vi "Actor Core.vi"(8 "error in":errorcluster, 11 "Sensor in":refnum<class "Sensor.lvclass">) -> (0 "error out":errorcluster, 3 "Actor out":refnum<class "Actor.lvclass">)   [LabVIEW 2012, in "Sensor Definition.lvlib" / "Sensor.lvclass"]
doc: "(<B>Filename</B>: Actor Framework.lvlib:Actor.lvclass:Actor Core.vi)\n\nReceives messages to the actor, reacts to them, and initiates any error handling that may shut the actor down.\n\nDescendant classes may override this VI to append parallel tasks for the actor to complete while it handles messages. Overrides use the Call Parent Method node."
uses:
  Sensor.lvclass
  <vilib>/ActorFramework/Actor/Actor.lvclass
  SensorCharm.lvclass
  Win8uiFramework/CharmView.lvclass
  <vilib>/ActorFramework/Actor/Actor.lvclass/Actor.ctl
  Sensor.lvclass/Sensor.ctl
  Write Owner.vi
  Read CharmView Actor.vi
  Write CharmView Actor.vi
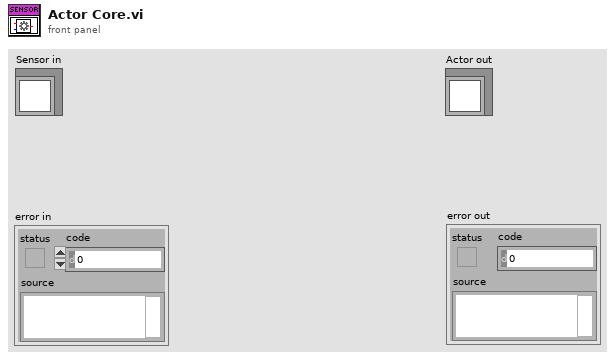
[diagram p1: front panel]
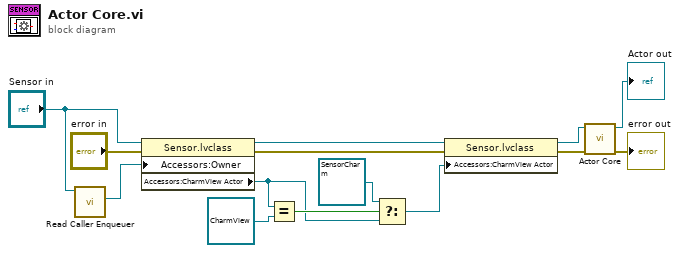
[diagram p0: block diagram]
diagram:
  n1 = call <vilib>:"Read Caller Enqueuer.vi"("Actor"="Sensor in") -> ("Caller Enqueuer"=w10:refnum<class "Message Enqueuer.lvclass">)  [unwired: 10 in]
  n2 = property class="Sensor.lvclass"(reference="Sensor in", error in="error in", "Accessors:Owner"=w10) -> (reference out=w9:refnum<class "Sensor.lvclass">, error out=w8:errorcluster, "Accessors:CharmView Actor"=w3:refnum<class "SensorCharm.lvclass">)
  n3 = Equal?(x=w3, y=refnum<class "CharmView.lvclass"> refnum ("Win8uiFramework.lvlib:CharmView.lvclass")) -> (x = y?=w4:bool)
  n4 = Select(t=refnum<class "SensorCharm.lvclass"> refnum ("Sensor Definition.lvlib:SensorCharm.lvclass"), s=w4, f=w3) -> (s? t:f=w1:refnum<class "SensorCharm.lvclass">)
  n5 = property class="Sensor.lvclass"(reference=w9, error in=w8, "Accessors:CharmView Actor"=w1) -> (reference out=w6:refnum<class "Sensor.lvclass">, error out=w7:errorcluster)
  n6 = call-parent "Actor Core.vi"("error in"=w7, "Actor in"=w6) -> ("error out"=→"error out":errorcluster, "Actor out"=→"Actor out":refnum<class "Actor.lvclass">)  [unwired: 8 in]
